vi "Totter.vi"(0 "Ultra_Sonic_Dist":dbl=inf, 2 "Level":bool=TRUE, 3 "Encoder":dbl=2664.99567, 5 "Auto_Enable":bool, 7 "Yaw":dbl=351.3276056000531, 9 "Auto_Selection":T2=enum."None", 11 "Extra_Dist":dbl, 12 "Stopped":bool=TRUE) -> (1 "Rest_Gyro":bool, 4 "TeeterTotter Enable":bool, 6 "Intake Arm Lowered":bool, 10 "Motor Speed":dbl, 14 "Rest_Encoder":bool, 15 "Completed_Auto":bool)   [LabVIEW 2015]
uses:
  Auto_Selection.ctl
  AutoEnum.ctl
  <vilib>/Rock Robotics/Network Tables/NT Read Number.vi
panel:
  in  "DB_Count":dbl=3.0
  in  "y":dbl=55.0
  in  "Drive Speed_2 Timeout":i32=10000
  in  "Drive_Speed_2":dbl=-1.0 format="%#_13g"
  in  "Drive_Speed_1_TIme out":i32=10000
  in  "Drive_one_Speed":dbl=-0.85 format="%#_13g"
  out "error":errorcluster
  out "State":T1
  in  "Dist_after_Totter":dbl=120.0
  in  "Dist to Tetter":dbl=41.0
  in  "Clear Error":bool
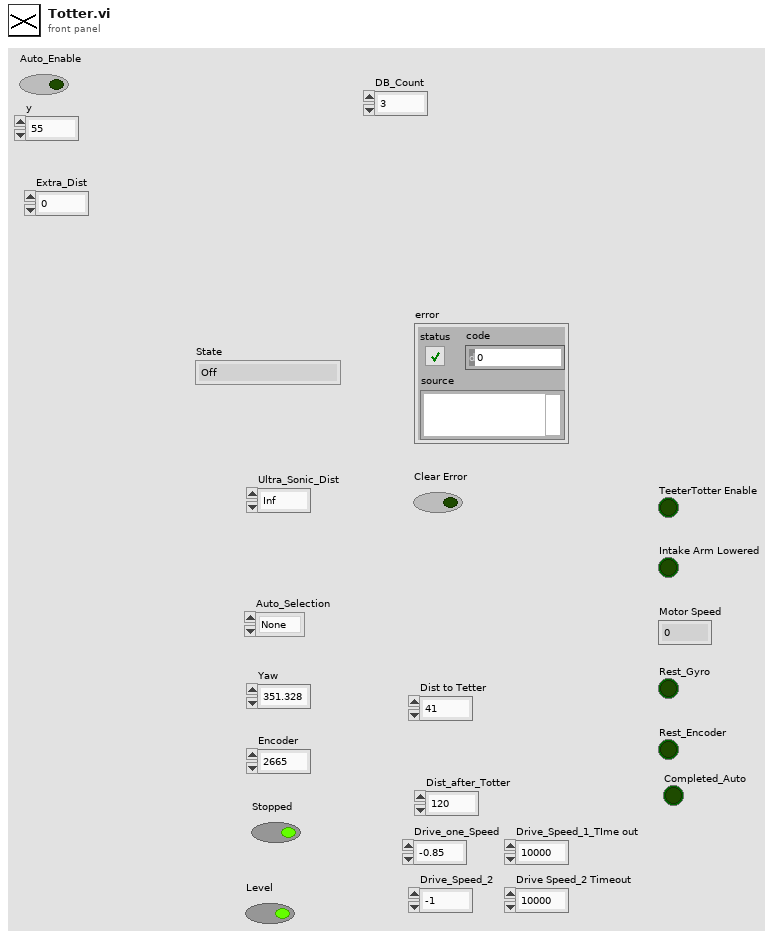
[diagram p1: front panel]
types:
  T1 = typedef "AutoEnum.ctl" = enum16{"Off", "ResetVar", "ResetOff", "BeforeTeeter", "LowerArm", "DriveForward", "Stop", "Stop One", "Drive Back", "Drive Forward Two"}
  T2 = typedef "Auto_Selection.ctl" = enum16{"Low Bar", "Rough Terrain", "Rock Wall", "Ramparts", "Moat", "Cheval de Frise", "Portcullis", "None", "One  Ball", "Shoot"}
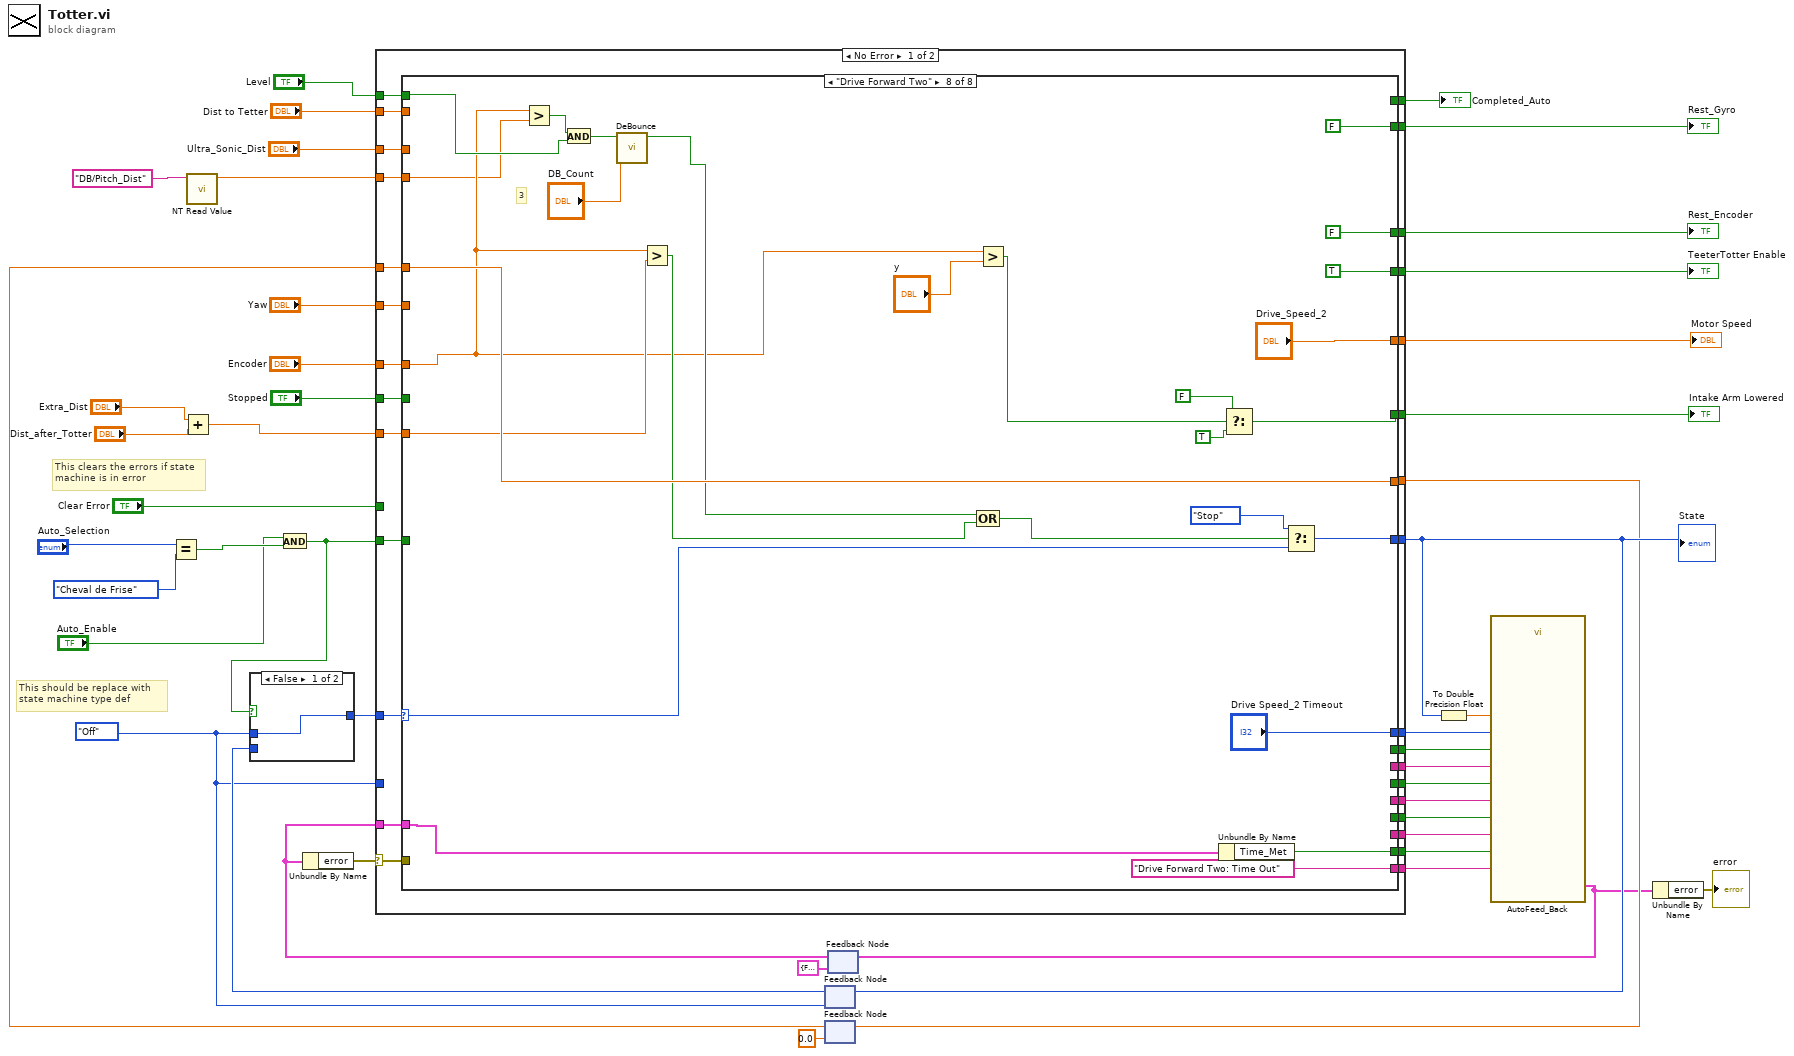
[diagram p0: block diagram]
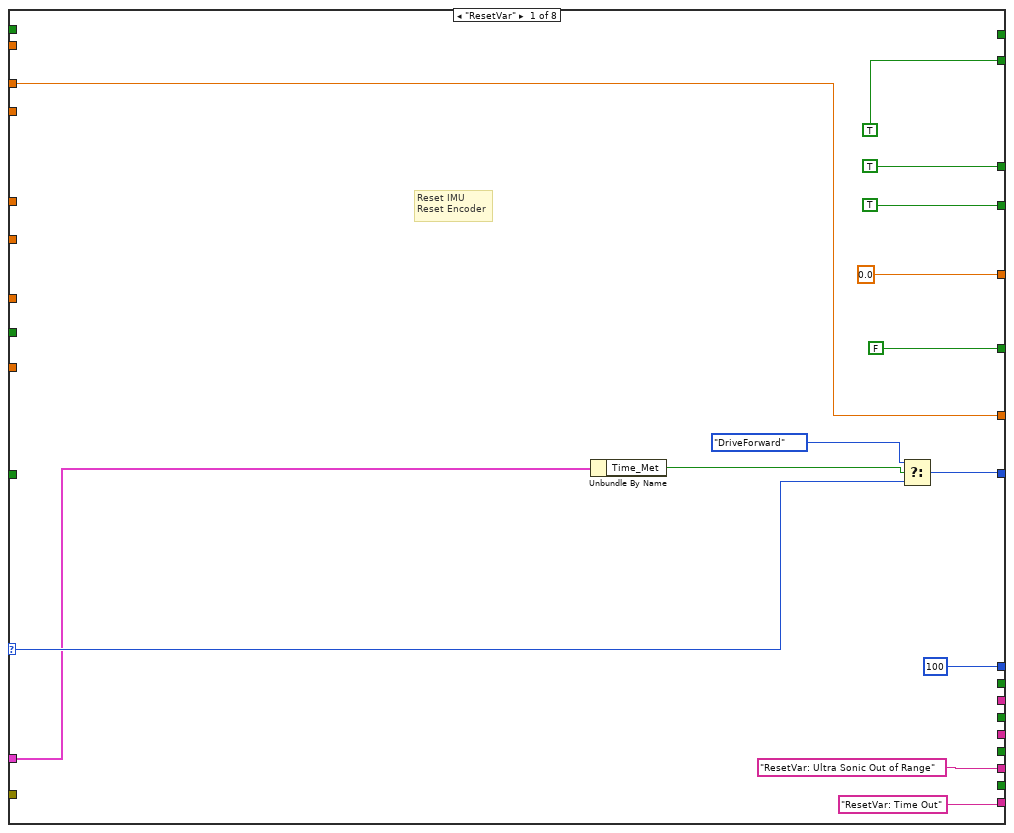
[diagram p3: hidden frame]
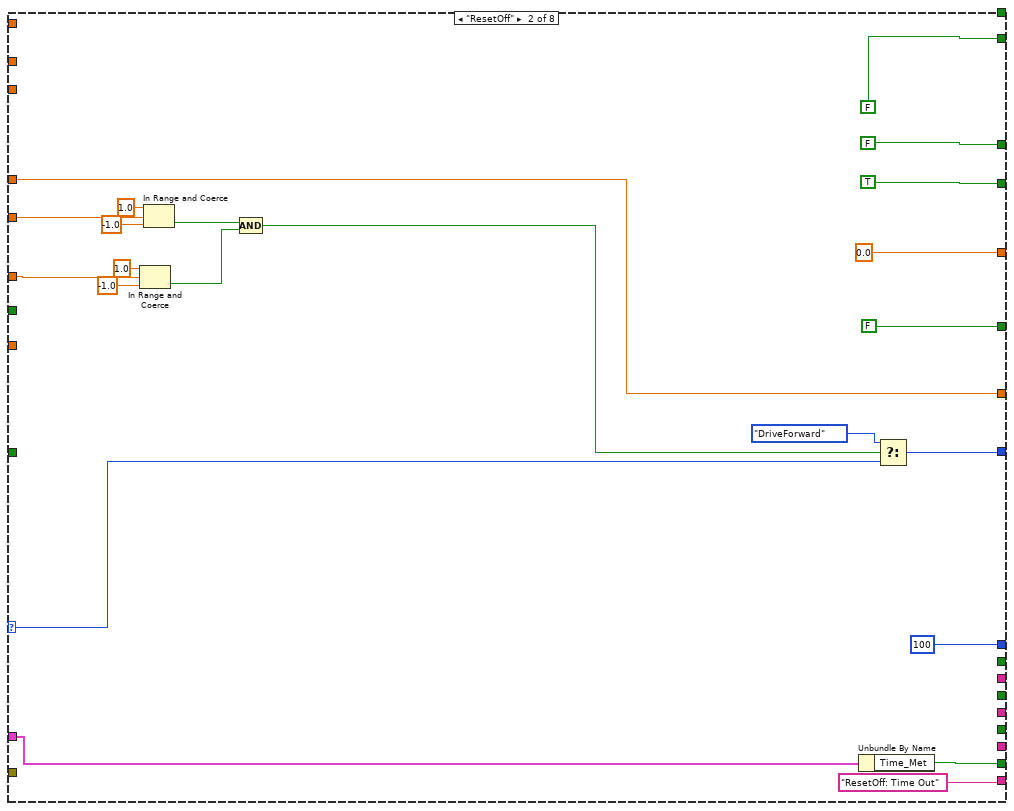
[diagram p4: hidden frame]
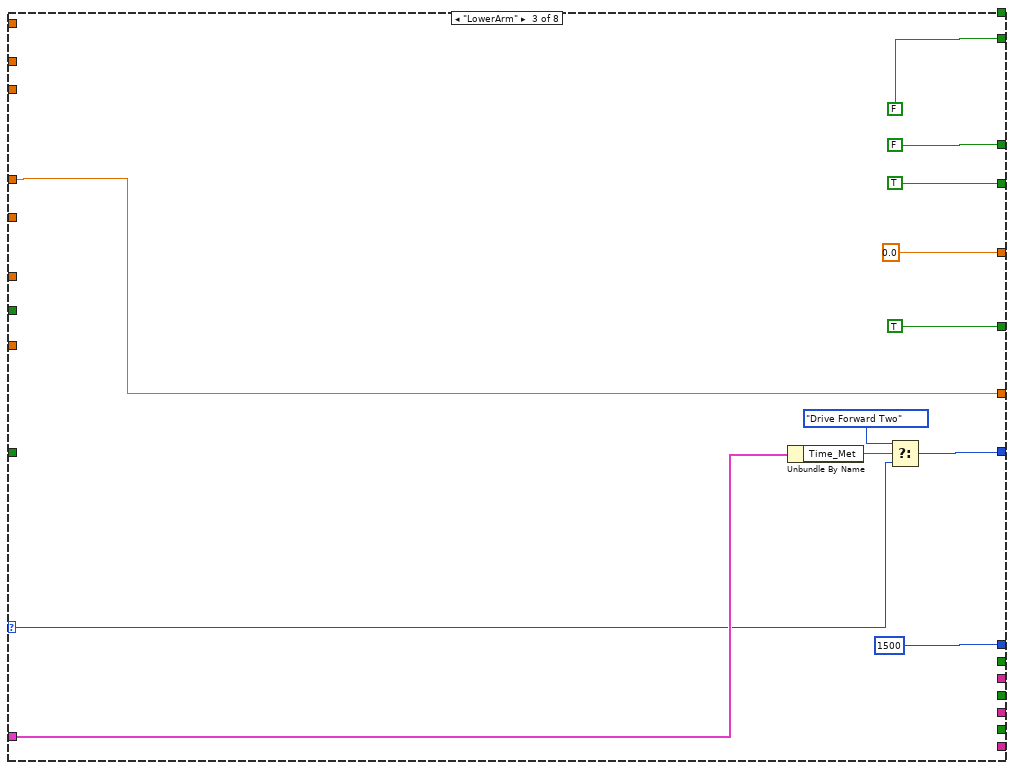
[diagram p5: hidden frame]
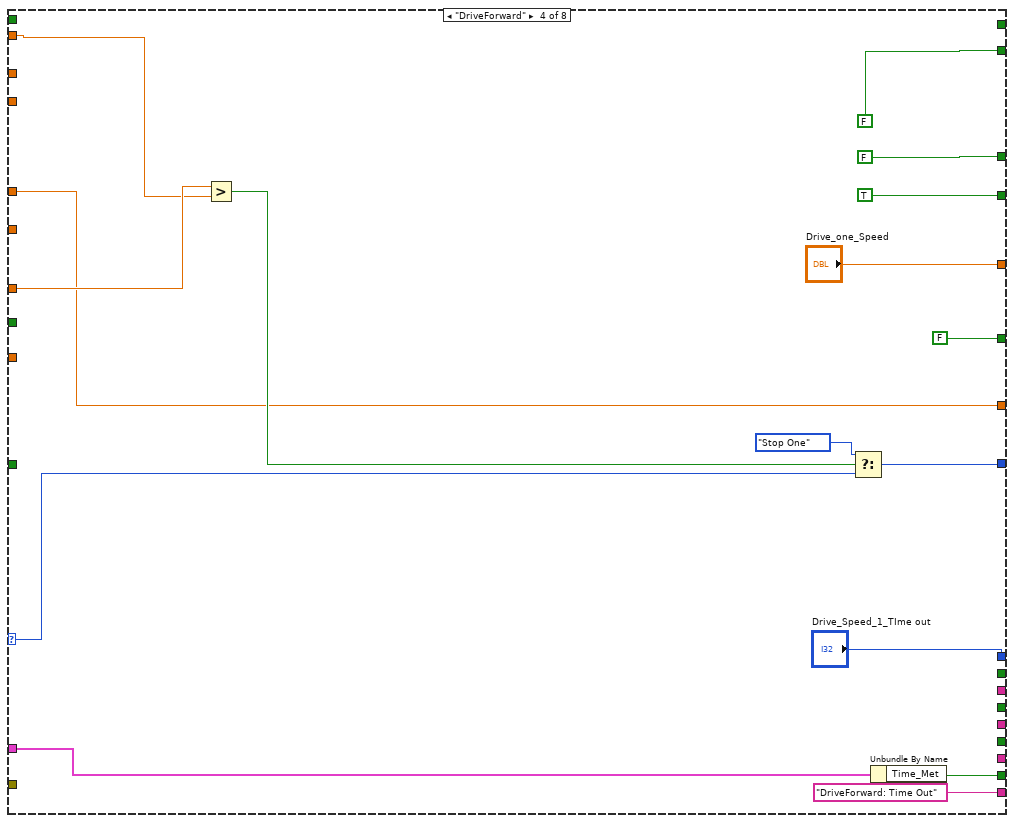
[diagram p6: hidden frame]
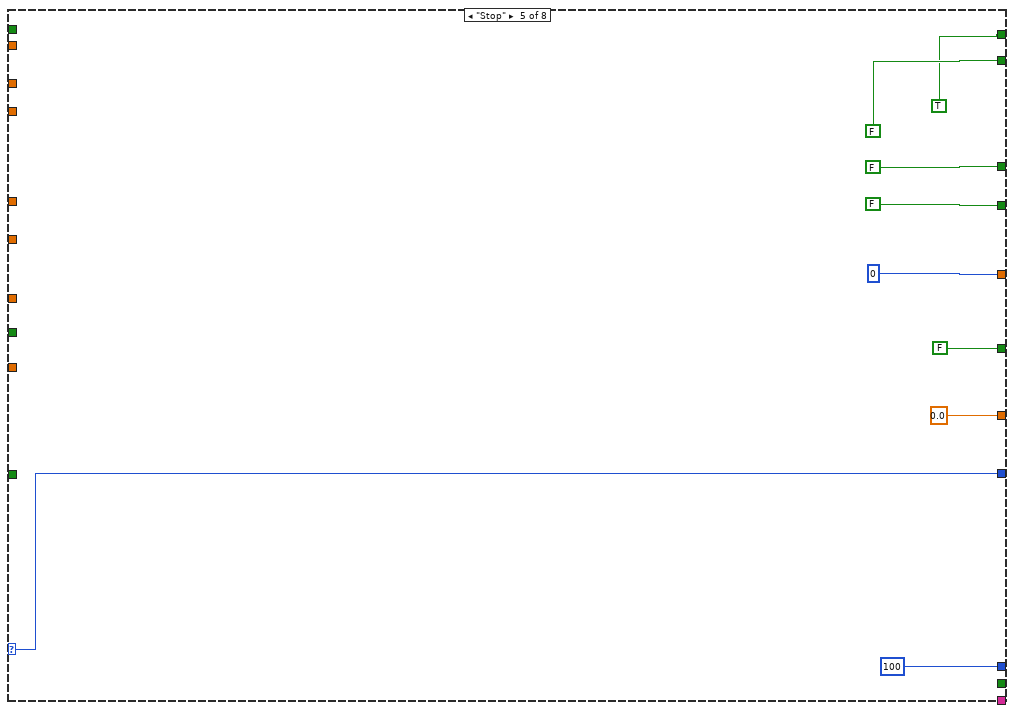
[diagram p7: hidden frame]
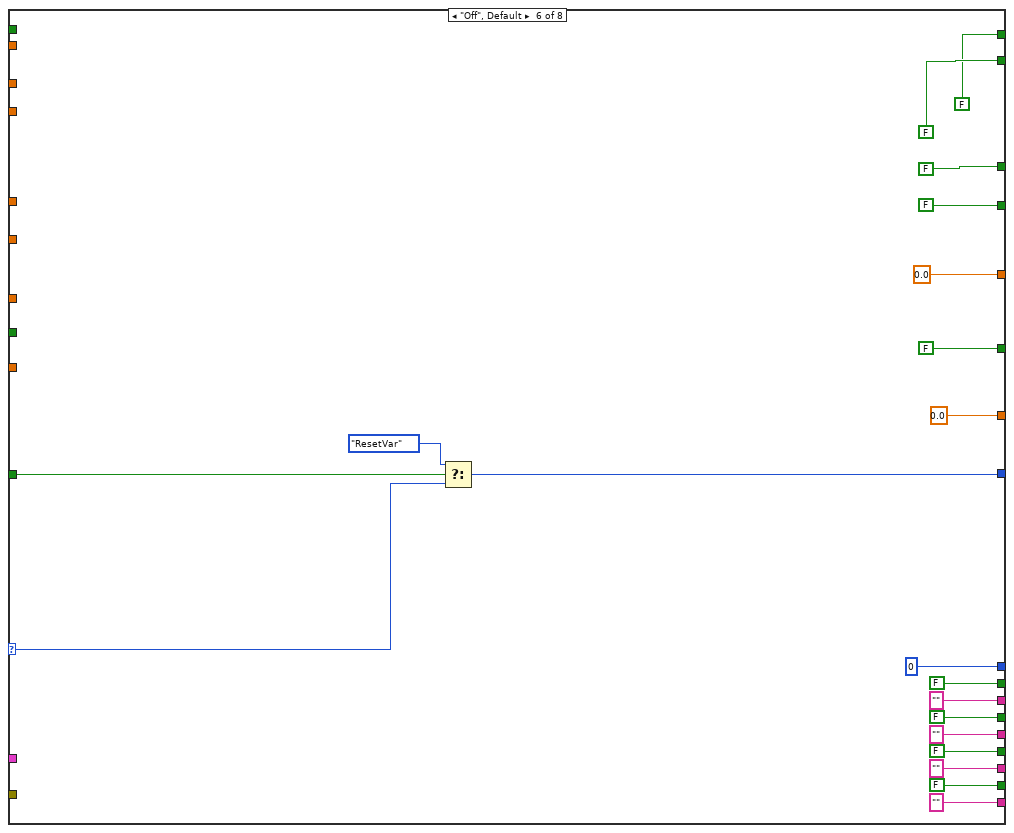
[diagram p8: hidden frame]
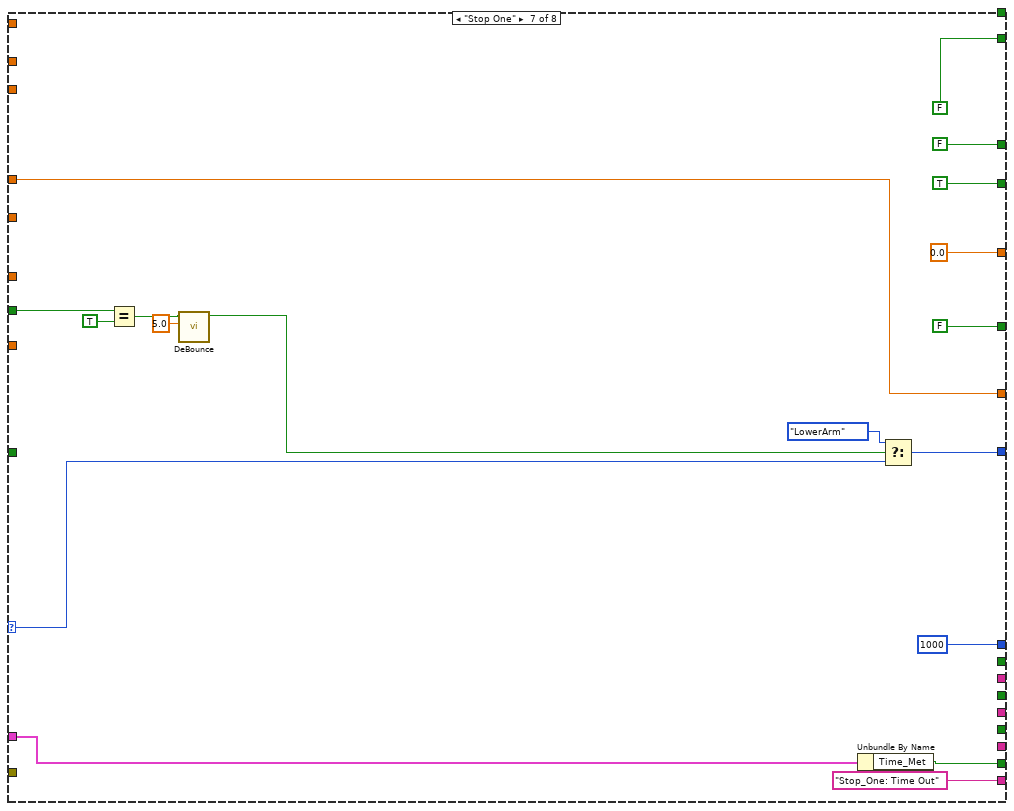
[diagram p9: hidden frame]
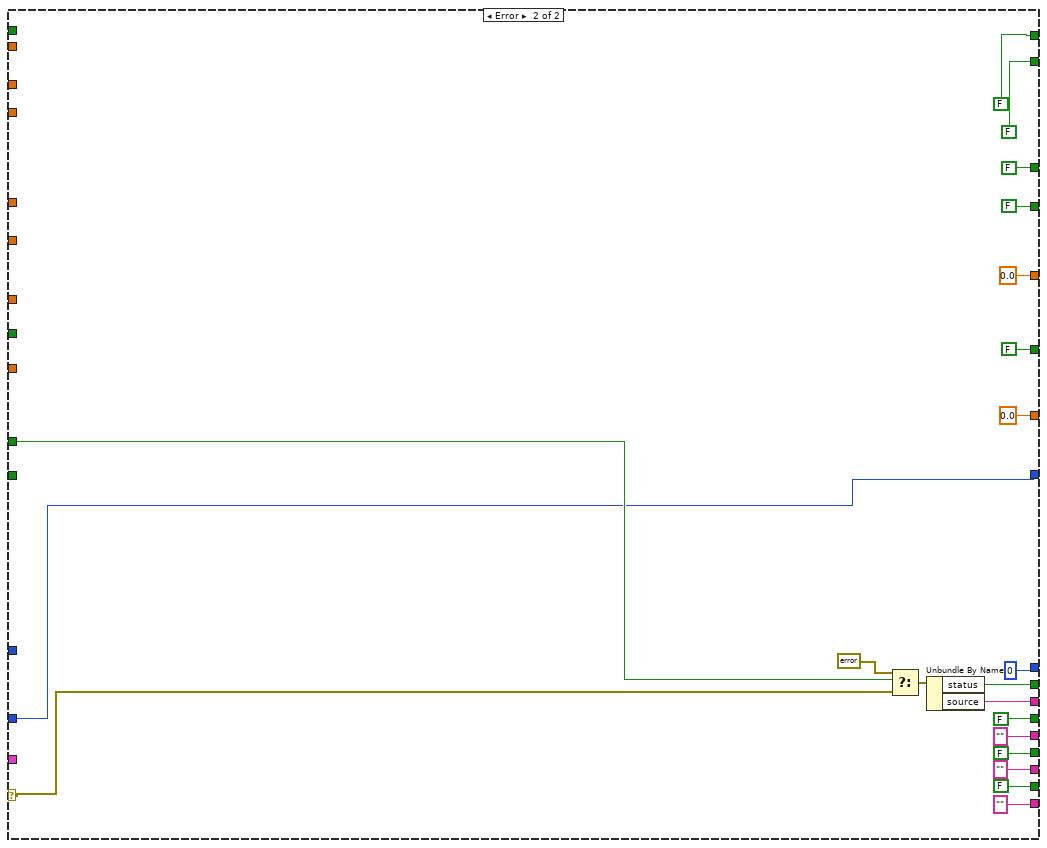
[diagram p10: hidden frame]
diagram:
  w36 = AutoEnum."Off"
  # "This clears the errors if state \nmachine is in error"
  # "This should be replace with \nstate machine type def"
  n1 = Equal?(x="Auto_Selection", y=Auto_Selection."Cheval de Frise" ("Auto_Selection")) -> (x = y?=w11:bool)
  n2 = Add(x="Extra_Dist", y="Dist_after_Totter") -> (x+y=w4:dbl)
  n3 = call-poly <vilib>:"NT Read Value.vi"("Name"="DB/Pitch_Dist" ("refnum name")) -> ("Numeric"=w1:dbl)  [unwired: 9 in, 1 out]
  n4 = And(x="Auto_Enable", y=w11) -> (x .and. y?=w8:bool)
  n5 = feedback #1(w36) -> (w38:T1)
  n6 = case shown="False" w8 {
    tunnel: w36 -> [w46 _]
    tunnel: [w46 w47] -> w39
    tunnel: w38 -> [_ w47]
    frame False {
    }
    frame True {
    }
  }
  n7 = feedback #2(0.0 ("Ultra_Sonic_Dist")) -> (w18:dbl)
  n8 = feedback #3(cluster{"Time_Met":bool, "error ":errorcluster} {"Time_Met"=FALSE, "error "={"status"=FALSE, "code"=0, "source"=""}} ("Feedback_State")) -> (w40:cluster{"Time_Met":bool, "error ":errorcluster})
  n9 = Unbundle By Name(w40) -> ("error"=w41:errorcluster)
  n10 = case shown="No Error" w41 {
    selector: w41 -> [w72 w233]
    tunnel: [w77 FALSE] -> w45
    tunnel: [w76 FALSE] -> w44
    tunnel: [w75 w217] -> w24
    tunnel: [w74 0] -> w43
    tunnel: "Clear Error" -> [_ w232]
    tunnel: w40 -> [w73 _]
    tunnel: w8 -> [w71 _]
    tunnel: w39 -> [w70 _]
    tunnel: w36 -> [_ w217]
    tunnel: [w69 0.0] -> w35
    tunnel: [w68 FALSE] -> w34
    tunnel: [w67 FALSE] -> w33
    tunnel: [w66 w220] -> w32
    tunnel: [w65 w219] -> w31
    tunnel: [w64 FALSE] -> w30
    tunnel: [w63 ""] -> w29
    tunnel: [w62 FALSE] -> w28
    tunnel: [w61 ""] -> w27
    tunnel: [w60 FALSE] -> w26
    tunnel: [w59 ""] -> w25
    tunnel: "Yaw" -> [w58 _]
    tunnel: "Encoder" -> [w57 _]
    tunnel: "Ultra_Sonic_Dist" -> [w56 _]
    tunnel: [w55 0.0 ("Ultra_Sonic_Dist")] -> w20
    tunnel: w18 -> [w54 _]
    tunnel: "Dist to Tetter" -> [w53 _]
    tunnel: "Stopped" -> [w52 _]
    tunnel: w4 -> [w51 _]
    tunnel: [w50 FALSE] -> w7
    tunnel: "Level" -> [w49 _]
    tunnel: w1 -> [w48 _]
    frame No Error {
      n11 = case shown="\"Drive Forward Two\"" w70 {
        selector: w70 -> [w83 w104 w114 w132 w143 w166 w183 w208]
        tunnel: [TRUE FALSE FALSE FALSE FALSE FALSE FALSE FALSE] -> w77
        tunnel: [TRUE FALSE FALSE FALSE FALSE FALSE FALSE FALSE] -> w76
        tunnel: [100 100 1500 "Drive_Speed_1_TIme out" 100 0 1000 "Drive Speed_2 Timeout"] -> w74
        tunnel: [w84 w107 w116 w135 w143 w165 w178 w210] -> w75
        tunnel: w73 -> [w79 w111 w119 w129 _ _ w180 w206]
        tunnel: w72 -> [_ _ _ _ _ _ _ _]
        tunnel: w71 -> [_ _ _ _ _ w167 _ _]
        tunnel: [0.0 0.0 0.0 "Drive_one_Speed" 0 0.0 0.0 "Drive_Speed_2"] -> w69
        tunnel: [TRUE TRUE TRUE TRUE FALSE FALSE TRUE TRUE] -> w68
        tunnel: [FALSE FALSE TRUE FALSE FALSE FALSE FALSE w198] -> w67
        tunnel: [_ _ _ _ _ FALSE _ _] -> w66
        tunnel: [_ _ _ _ _ "" _ _] -> w65
        tunnel: [_ _ _ _ _ FALSE _ _] -> w64
        tunnel: [_ _ _ _ _ "" _ _] -> w63
        tunnel: [_ _ _ _ _ FALSE _ _] -> w62
        tunnel: ["ResetVar: Ultra Sonic Out of Range" _ _ _ _ "" _ _] -> w61
        tunnel: [_ w106 _ w128 _ FALSE w171 w205] -> w60
        tunnel: ["ResetVar: Time Out" "ResetOff: Time Out" _ "DriveForward: Time Out" _ "" "Stop_One: Time Out" "Drive Forward Two: Time Out"] -> w59
        tunnel: w58 -> [_ w103 _ _ _ _ _ _]
        tunnel: w57 -> [_ w98 _ w136 _ _ _ w190]
        tunnel: w56 -> [w81 _ _ _ _ _ _ _]
        tunnel: [w81 w92 w115 w130 0.0 ("Ultra_Sonic_Dist") 0.0 ("Ultra_Sonic_Dist") w172 w211] -> w55
        tunnel: w54 -> [_ w92 w115 w130 _ _ w172 w211]
        tunnel: w53 -> [_ _ _ w126 _ _ _ _]
        tunnel: w52 -> [_ _ _ _ _ _ w188 _]
        tunnel: w51 -> [_ _ _ _ _ _ _ w203]
        tunnel: [_ _ _ _ TRUE FALSE _ _] -> w50
        tunnel: w49 -> [_ _ _ _ _ _ _ w191]
        tunnel: w48 -> [_ _ _ _ _ _ _ w189]
        frame "ResetVar" {
          # "Reset IMU\nReset Encoder"
          n12 = Unbundle By Name(w79) -> ("Time_Met"=w78:bool)
          n13 = Select(t=AutoEnum."DriveForward", s=w78, f=w83) -> (s? t:f=w84:T1)
        }
        frame "ResetOff" {
          n14 = In Range and Coerce(upper limit=1.0, x=w98, lower limit=-1.0) -> (In Range?=w96:bool)  [unwired: 1 out]
          n15 = In Range and Coerce(upper limit=1.0, x=w103, lower limit=-1.0) -> (In Range?=w97:bool)  [unwired: 1 out]
          n16 = Compound Arithmetic op=AND(w97, w96) -> (w95:bool)
          n17 = Unbundle By Name(w111) -> ("Time_Met"=w106:bool)
          n18 = Select(t=AutoEnum."DriveForward", s=w95, f=w104) -> (s? t:f=w107:T1)
        }
        frame "LowerArm" {
          n19 = Unbundle By Name(w119) -> ("Time_Met"=w121:bool)
          n20 = Select(t=AutoEnum."Drive Forward Two", s=w121, f=w114) -> (s? t:f=w116:T1)
        }
        frame "DriveForward" {
          n21 = Greater?(x=w136, y=w126) -> (0:w134:bool)
          n22 = Select(t=AutoEnum."Stop One", s=w134, f=w132) -> (s? t:f=w135:T1)
          n23 = Unbundle By Name(w129) -> ("Time_Met"=w128:bool)
        }
        frame "Stop" {
        }
        frame "Off", Default {
          n24 = Select(t=AutoEnum."ResetVar", s=w167, f=w166) -> (s? t:f=w165:T1)
        }
        frame "Stop One" {
          n25 = Equal?(x=w188, y=TRUE) -> (x = y?=w186:bool)
          n26 = call "DeBounce.vi"("DB_Count"=5.0, "Value"=w186) -> ("BD_Value"=w184:bool)  [unwired: 9 in]
          n27 = Unbundle By Name(w180) -> ("Time_Met"=w171:bool)
          n28 = Select(t=AutoEnum."LowerArm", s=w184, f=w183) -> (s? t:f=w178:T1)
        }
        frame "Drive Forward Two" {
          # "3"
          n29 = Greater?(x=w190, y=w189) -> (0:w193:bool)
          n30 = And(x=w193, y=w191) -> (x .and. y?=w194:bool)
          n31 = call "DeBounce.vi"("DB_Count"="DB_Count", "Value"=w194) -> ("BD_Value"=w192:bool)  [unwired: 9 in]
          n32 = Greater?(x=w190, y=w203) -> (0:w197:bool)
          n33 = Compound Arithmetic op=OR(w192, w197) -> (w196:bool)
          n34 = Greater?(x=w190, y="y") -> (0:w201:bool)
          n35 = Unbundle By Name(w206) -> ("Time_Met"=w205:bool)
          n36 = Select(t=FALSE, s=w201, f=TRUE) -> (s? t:f=w198:bool)
          n37 = Select(t=AutoEnum."Stop", s=w196, f=w208) -> (s? t:f=w210:T1)
        }
      }
    }
    frame Error {
      n38 = Select(t=errorcluster {"status"=FALSE, "code"=0, "source"=""}, s=w232, f=w233) -> (s? t:f=w221:errorcluster)
      n39 = Unbundle By Name(w221) -> ("status"=w220:bool, "source"=w219:string)
    }
  }
  "Rest_Gyro" <- w45
  "Rest_Encoder" <- w44
  "Motor Speed" <- w35
  "TeeterTotter Enable" <- w34
  "Intake Arm Lowered" <- w33
  "State" <- w24
  "Completed_Auto" <- w7
  n40 = feedback-in #1(w24) -> ()
  n41 = feedback-in #2(w20) -> ()
  n42 = To Double Precision Float(number=w24) -> (double precision float=w37:dbl)
  n43 = call "AutoFeed_Back.vi"("Code 4"=w25, "Error_4_En"=w26, "Code 3"=w27, "Code 2"=w29, "Error_3_En"=w28, "Error_2_En"=w30, "Code 1"=w31, "Error_1_En"=w32, "Time (ms)"=w43, "State"=w37) -> ("Feedback_State"=w13:cluster{"Time_Met":bool, "error ":errorcluster})  [unwired: 1 in]
  n44 = feedback-in #3(w13) -> ()
  n45 = Unbundle By Name(w13) -> ("error"=→"error":errorcluster)
